vi "WPI_CameraSet Color Enable.vi"(8 "error in (no error)":errorcluster, 10 "Color Enabled":bool, 11 "CameraDevRef":T1={"Camera Address"="192.168.0.90", "CameraStatus"={"status"=FALSE, "code"=0, "source"=""}}) -> (0 "error out":errorcluster, 3 "CameraDevRef Out":T1)   [LabVIEW 2017]
doc: "Determine whether the images from the camera are encoded in color or grayscale. Grayscale images are smaller in size, and may simplify processing in some circumstances.\n\nThis software is licensed. Open the labview\\readme\\WPI Robotics Library Open Source License.txt file for more information."
uses:
  <vilib>/Rock Robotics/WPI/Camera/WPI_CameraDevRef.ctl
  <vilib>/Rock Robotics/WPI/Camera/WPI_CameraSettings Operations.ctl
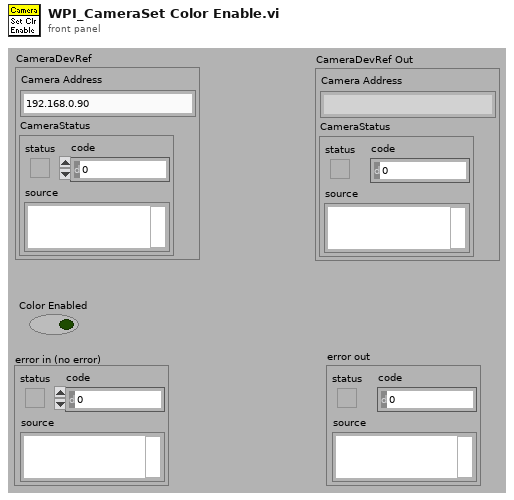
[diagram p1: front panel]
types:
  T1 = typedef "WPI_CameraDevRef.ctl" = cluster{"Camera Address":string, "CameraStatus":errorcluster}
  T2 = typedef "WPI_CameraSettings Operations.ctl" = enum16{"Udate FPS", "Update Compression", "Update Size", "Update White Balance", "Update Brightness", "Update Sharpness", "Update Exposure", "Update Exposure Value", "Update Color Level", "Update Exp Priority", "Update Color Enable", "Update JPG", "Update MJPG", "Read and Clear", "Read", "Init"}
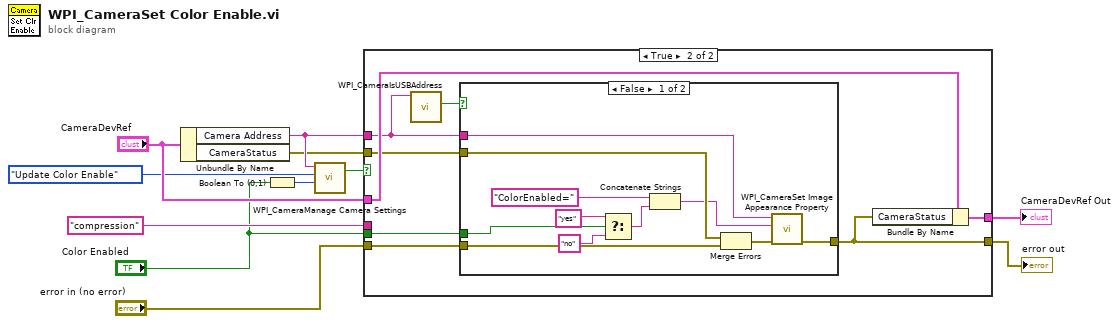
[diagram p0: block diagram]
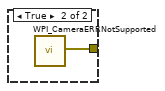
[diagram p3: hidden frame]
diagram:
  n1 = Unbundle By Name("CameraDevRef") -> ("Camera Address"=w4:string, "CameraStatus"=w3:errorcluster)
  n2 = Boolean To (0,1)(Boolean="Color Enabled") -> (0, 1=w2:i16)
  n3 = call <vilib>:"WPI_CameraManage Camera Settings.vi"("Value"=w2, "Operation"=WPI_CameraSettings_Operations."Update Color Enable", "Camera IP"=w4) -> ("Changed"=w9:bool)  [unwired: 7 in, 1 out]
  n4 = case shown="True" w9 {
    tunnel: "CameraDevRef" -> [w12 w19]
    tunnel: "compression" ("Property Name") -> [_ _]
    tunnel: "Color Enabled" -> [_ w16]
    tunnel: [w12 w20] -> w10
    tunnel: "error in (no error)" -> [w13 w18]
    tunnel: [w13 w21] -> w5
    tunnel: w4 -> [_ w15]
    tunnel: w3 -> [_ w17]
    frame False {
    }
    frame True {
      n5 = call <vilib>:"WPI_CameraIsUSBAddress.vi"("Camera Address In"=w15) -> ("USB?"=w14:bool)  [unwired: 8 in, 2 out]
      n6 = case shown="False" w14 {
        tunnel: [w32 w33] -> w21
        tunnel: w18 -> [w31 _]
        tunnel: w17 -> [w29 _]
        tunnel: w16 -> [w23 _]
        tunnel: w15 -> [w22 _]
        frame False {
          n7 = Select(t="yes" ("Property Name"), s=w23, f="no" ("Property Name")) -> (s? t:f=w28:string)
          n8 = Concatenate Strings("ColorEnabled=" ("Property Name"), w28) -> (w24:string)
          n9 = Merge Errors(w29, w31) -> (w30:errorcluster)
          n10 = call <vilib>:"WPI_CameraSet Image Appearance Property.vi"("error in"=w30, "Prop String"=w24, "address"=w22) -> ("error out"=w32:errorcluster)  [unwired: 1 in, 7 out]
        }
        frame True {
          n11 = call <vilib>:"WPI_CameraERRNotSupported.vi"() -> ("error out"=w33:errorcluster)
        }
      }
      n12 = Bundle By Name(cluster=w19, "CameraStatus"=w21) -> (w20:T1)
    }
  }
  "CameraDevRef Out" <- w10
  "error out" <- w5
